vi "rotated_picture_init.vi"(11 "Picture FIle Name":string) -> (0 "Six-colors":u32[](array[numeric]), 1 "Five-Numeric 3":cdb, 2 "Four-Numeric":i32, 3 "Three-Numeric 2":i32, 4 "Seven-new element/subarray":u32, 5 "Two-Array":cdb[][](array[numeric]), 6 "Eight-Cluster":cluster{"[0]":i32, "[1]":i32}, 7 "ONE-8-bit pixmap":u8[][](array[numeric]))   [LabVIEW 2019]
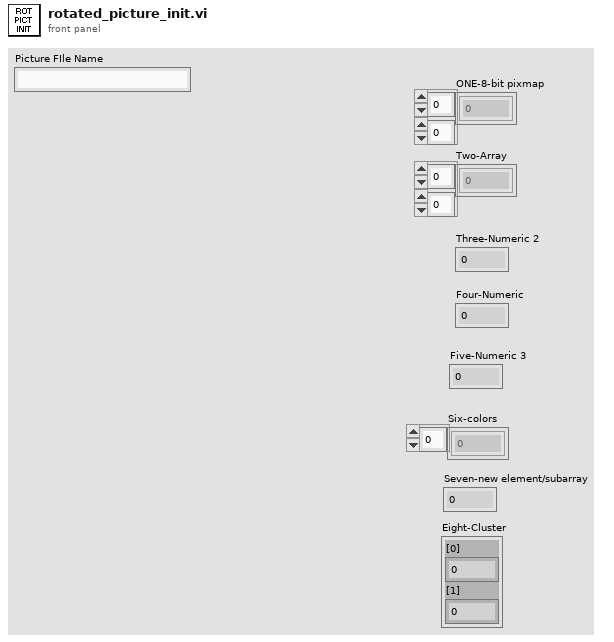
[diagram p1: front panel]
types:
  T1 = typedef "imagedata.ctl" = cluster{"image type":i32, "image depth":i32, "image":u8[], "mask":u8[], "colors":u32[], "Rectangle":cluster{"left":i16, "top":i16, "right":i16, "bottom":i16}}
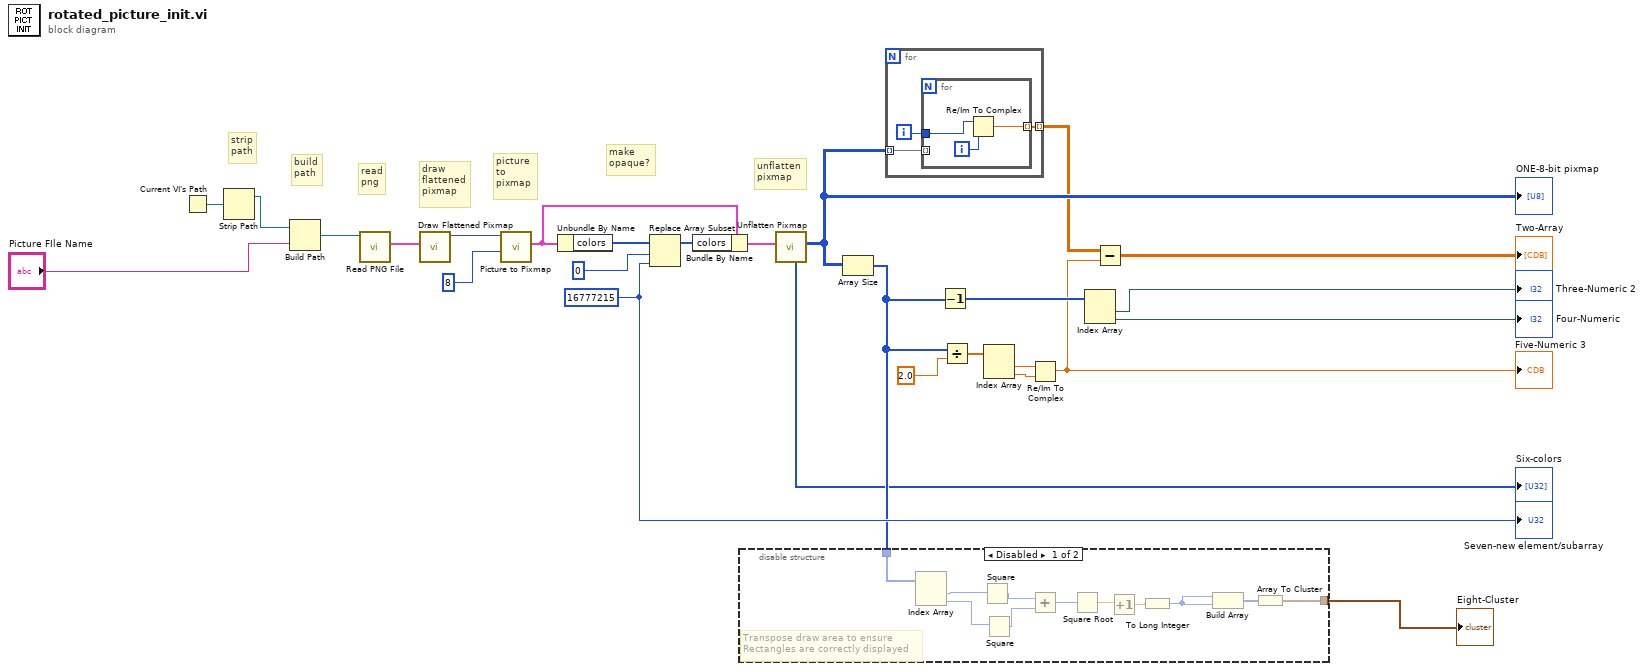
[diagram p0: block diagram]
diagram:
  w26 = u32 16777215 ("new element/subarray")
  # "unflatten\npixmap"
  # "make\nopaque?"
  # "picture\nto\npixmap"
  # "draw\nflattened\npixmap"
  # "read\npng"
  # "build\npath"
  # "strip\npath"
  n1 = Current VI's Path() -> (path=w12:path)
  n2 = Strip Path(path=w12) -> (stripped path=w15:path)  [unwired: 1 out]
  n3 = Build Path(base path=w15, name or relative path="Picture FIle Name") -> (appended path=w13:path)
  n4 = call <vilib>:"Read PNG File.vi"("path to PNG file"=w13) -> ("image data"=w21:T1)  [unwired: 8 in, 2 out]
  n5 = call <vilib>:"Draw Flattened Pixmap.vi"("image data"=w21) -> ("new picture"=w22:picture)  [unwired: 8 in]
  n6 = call <vilib>:"Picture to Pixmap.vi"("depth"=8, "picture"=w22) -> ("image data"=w24:T1)  [unwired: 8 in, 1 out]
  n7 = Unbundle By Name(w24) -> ("colors"=w18:u32[])
  n8 = Replace Array Subset(array=w18, new element=w26, index=0) -> (w20:u32[])
  n9 = Bundle By Name(cluster=w24, "colors"=w20) -> (w25:T1)
  n10 = call <vilib>:"Unflatten Pixmap.vi"("image data"=w25) -> ("8-bit pixmap"=w17:u8[][], "colors"=→"Six-colors":u32[])  [unwired: 4 in, 5 out]
  "ONE-8-bit pixmap" <- w17
  n11 = Array Size(array=w17) -> (size(s)=w16:i32[])
  n12 = disable-structure shown="Disabled" {
    disable-tunnel: w16 -> [w38 _]
    disable-tunnel: [w28 _] -> w27
    frame Disabled {
      # "Transpose draw area to ensure \nRectangles are correctly displayed"
      n13 = Index Array(array=w38) -> (element #1=w37:i32, element #2=w36:i32)  [unwired: 2 in]
      n14 = Square(x=w37) -> (x^2=w35:i32)
      n15 = Square(x=w36) -> (x^2=w34:i32)
      n16 = Add(x=w35, y=w34) -> (x+y=w33:i32)
      n17 = Square Root(x=w33) -> (sqrt(x)=w32:dbl)
      n18 = Increment(x=w32) -> (x+1=w31:dbl)
      n19 = To Long Integer(number=w31) -> (32bit integer=w30:i32)
      n20 = Build Array(w30, w30) -> (w29:i32[])
      n21 = Array To Cluster(array=w29) -> (cluster=w28:cluster{"[0]":i32, "[1]":i32})
    }
    frame Enabled {
    }
  }
  "Eight-Cluster" <- w27
  n22 = for {
    tunnel: [w40] -> w1 mode=indexing
    tunnel: w17 -> [w39] mode=indexing
    i -> [w41]
    n23 = for {
      tunnel: w41 -> [w44]
      tunnel: [w43] -> w40 mode=indexing
      tunnel: w39 -> [_] mode=indexing
      i -> [w42]
      n24 = Re/Im To Complex(1:w42, 2:w44) -> (0:w43:cdb)
    }
  }
  n25 = Decrement(x=w16) -> (x-1=w11:i32[])
  n26 = Divide(x=w16, y=2.0) -> (x/y=w5:dbl[])
  n27 = Index Array(array=w5) -> (element #1=w7:dbl, element #2=w8:dbl)  [unwired: 2 in]
  n28 = Re/Im To Complex(1:w8, 2:w7) -> (0:w3:cdb)
  "Five-Numeric 3" <- w3
  n29 = Index Array(array=w11) -> (element #1=→"Three-Numeric 2":i32, element #2=→"Four-Numeric":i32)  [unwired: 2 in]
  n30 = Subtract(x=w1, y=w3) -> (x-y=→"Two-Array":cdb[][])
  "Seven-new element/subarray" <- w26
